vi "Write.vi"(8 "error in":errorcluster, 10 "PCAN Message":T2 {"DATA"."7" format="%.0x"; "DATA"."6" format="%.0x"; "DATA"."5" format="%.0x"; "DATA"."4" format="%.0x"; "DATA"."3" format="%.0x"; "DATA"."2" format="%.0x"; "DATA"."1" format="%.0x"; "DATA"."0" format="%.0x"; "MSGTYPE" items=["STANDARD"=0, "RTR"=1, "EXTENDED"=2, "FD"=4, "BRS"=8, "ESI"=16, "ECHO"=32, "ERRFRAME"=64, "STATUS"=128]}, 11 "TPCANHandle in":T1=81 items=["PCAN_NONEBUS"=0, "PCAN_USBBUS1"=81, "PCAN_USBBUS2"=82, "PCAN_USBBUS3"=83, "PCAN_USBBUS4"=84, "PCAN_USBBUS5"=85, "PCAN_USBBUS6"=86, "PCAN_USBBUS7"=87, "PCAN_USBBUS8"=88, "PCAN_USBBUS9"=1289, "PCAN_USBBUS10"=1290, "PCAN_USBBUS11"=1291, "PCAN_USBBUS12"=1292, "PCAN_USBBUS13"=1293, "PCAN_USBBUS14"=1294, "PCAN_USBBUS15"=1295, "PCAN_USBBUS16"=1296]) -> (0 "error out":errorcluster, 3 "TPCANHandle out":T1=81 items=["PCAN_NONEBUS"=0, "PCAN_USBBUS1"=81, "PCAN_USBBUS2"=82, "PCAN_USBBUS3"=83, "PCAN_USBBUS4"=84, "PCAN_USBBUS5"=85, "PCAN_USBBUS6"=86, "PCAN_USBBUS7"=87, "PCAN_USBBUS8"=88, "PCAN_USBBUS9"=1289, "PCAN_USBBUS10"=1290, "PCAN_USBBUS11"=1291, "PCAN_USBBUS12"=1292, "PCAN_USBBUS13"=1293, "PCAN_USBBUS14"=1294, "PCAN_USBBUS15"=1295, "PCAN_USBBUS16"=1296], 5 "TPCANStatus":T4 items=["PCAN_ERROR_OK"=0, "PCAN_ERROR_XMTFULL"=1, "PCAN_ERROR_OVERRUN"=2, "PCAN_ERROR_BUSLIGHT"=4, "PCAN_ERROR_BUSHEAVY"=8, "PCAN_ERROR_BUSPASSIVE"=262144, "PCAN_ERROR_BUSOFF"=16, "PCAN_ERROR_QRCVEMPTY"=32, "PCAN_ERROR_QOVERRUN"=64, "PCAN_ERROR_QXMTFULL"=128, "PCAN_ERROR_REGTEST"=256, "PCAN_ERROR_NODRIVER"=512, "PCAN_ERROR_HWINUSE"=1024, "PCAN_ERROR_NETINUSE"=2048, "PCAN_ERROR_ILLHW"=5120, "PCAN_ERROR_ILLNET"=6144, "PCAN_ERROR_ILLCLIENT"=7168, "PCAN_ERROR_RESOURCE"=8192, "PCAN_ERROR_ILLPARAMTYPE"=16384, "PCAN_ERROR_ILLPARAMVAL"=32768, "PCAN_ERROR_UNKNOWN"=65536, "PCAN_ERROR_ILLDATA"=131072, "PCAN_ERROR_ILLMODE"=524288, "PCAN_ERROR_CAUTION"=33554432, "PCAN_ERROR_INITIALIZE"=67108864, "PCAN_ERROR_ILLOPERATION"=134217728])   [LabVIEW 2018, in "PCANBasic.lvlib"]
doc: "Transmits a CAN message.\nIf a bus-off error occur, an application cannot use the channel to communicate anymore, until the CAN controller is reset. With PCAN-Basic it is not possible to reset the CAN controller through a method directly. Consider using the PCAN-Basic property PCAN_BUSOFF_AUTORESET which instructs the API to automatically reset the CAN controller when a bus-off state is detected. \n\nAnother ways to reset errors like bus-off, bus-heavy and bus-light:\n\nPerforming an uninitialize / initialize cycle: This causes a hardware reset, but only when no more clients are connected to that channel. \nUsing the parameter PCAN_HARD_RESET_STATUS: It instructs this method to explicitly perform a hardware reset regardless of whether other clients are connected to that channel."
uses:
  PCANBasic.lvlib
  TPCANHandle.ctl
  PCAN Message types.ctl
  PCAN Message.ctl
  TPCANStatus.ctl
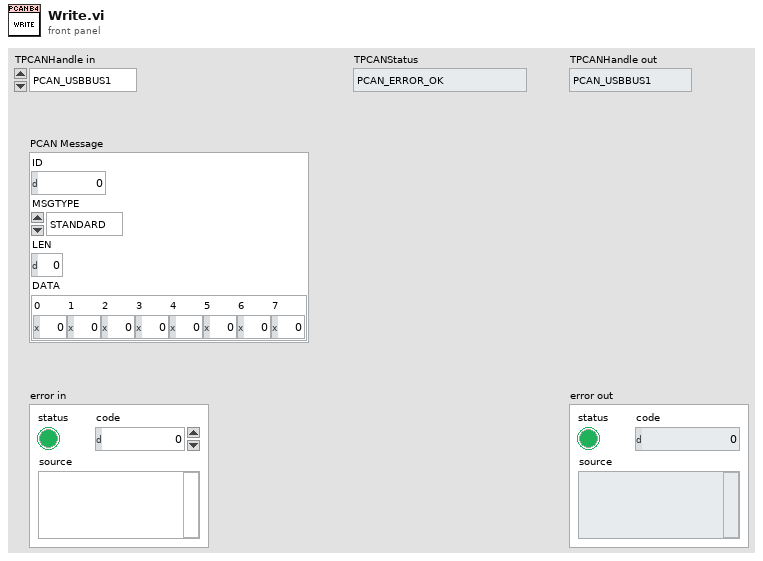
[diagram p1: front panel]
types:
  T1 = typedef "PCANBasic.lvlib/TPCANHandle.ctl" = u16
  T2 = typedef "PCANBasic.lvlib/PCAN Message.ctl" = cluster{"ID":u32, "MSGTYPE":T3, "LEN":u8, "DATA":cluster{"0":u8, "1":u8, "2":u8, "3":u8, "4":u8, "5":u8, "6":u8, "7":u8}}
  T3 = typedef "PCANBasic.lvlib/PCAN Message types.ctl" = u8
  T4 = typedef "PCANBasic.lvlib/TPCANStatus.ctl" = u32
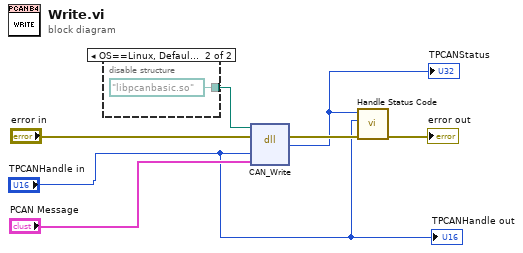
[diagram p0: block diagram]
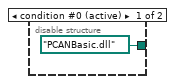
[diagram p2: hidden frame]
diagram:
  n1 = disable-structure shown="OS==Linux, Default" {
    disable-tunnel: [path "PCANBasic.dll" path "libpcanbasic.so"] -> w2
    frame condition #0 (active) {
    }
    frame condition #1 {
    }
  }
  n2 = dll-call lib="?" fn="CAN_Write"(path in=w2, error in="error in", "Channel"="TPCANHandle in", "MessageBuffer"="PCAN Message") -> (error out=w5:errorcluster, "TPCANStatus"=w4:u32)  [unwired: 3 in, 1 out]
  "TPCANStatus" <- w4
  n3 = call "Handle Status Code.vi"("error in"=w5, "TPCANHandle"="TPCANHandle in", "TPCANStatus"=w4) -> ("error out"=→"error out":errorcluster)  [unwired: 8 in]
  "TPCANHandle out" <- "TPCANHandle in"
